vi "Dim2Name.vi"(10 "StackedAvg":u16[][][](array[numeric]), 11 "name":string) -> (3 "String":string)   [LabVIEW 2014]
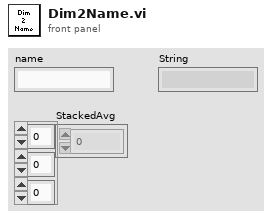
[diagram p1: front panel]
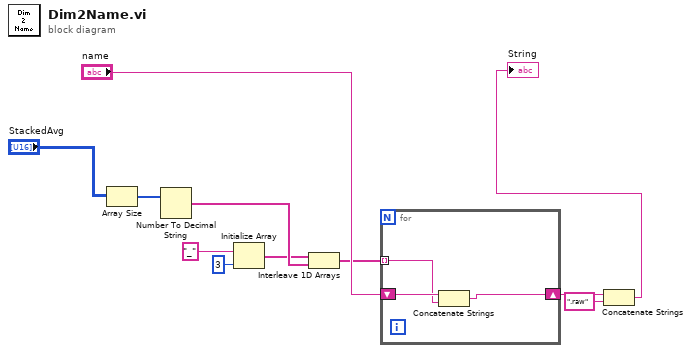
[diagram p0: block diagram]
diagram:
  n1 = Array Size(array="StackedAvg") -> (size(s)=w2:i32[])
  n2 = Number To Decimal String(number=w2) -> (decimal integer string=w6:string[])  [unwired: 1 in]
  n3 = Initialize Array("_", 3 ("dimension size")) -> (w5:string[])
  n4 = Interleave 1D Arrays(w5, w6) -> (w7:string[])
  n5 = for {
    tunnel: w7 -> [w13] mode=indexing
    shift-right: [w12] -> w9
    shift-left: "name" -> [w14]
    n6 = Concatenate Strings(w14, w13) -> (w12:string)
  }
  n7 = Concatenate Strings(w9, ".raw" ("string")) -> (→"String":string)
